vi "DEMO.vi"(8 "errin":errorcluster, 10 "DATA IN":T1) -> (0 "error out":errorcluster)   [LabVIEW 2020]
uses:
  93f8419f-589b-4a81-b62e-70ffcd900bdb.vi
  OP600/SubVI/CheminDeBase.vi
panel:
  out "chaîne concaténée":string
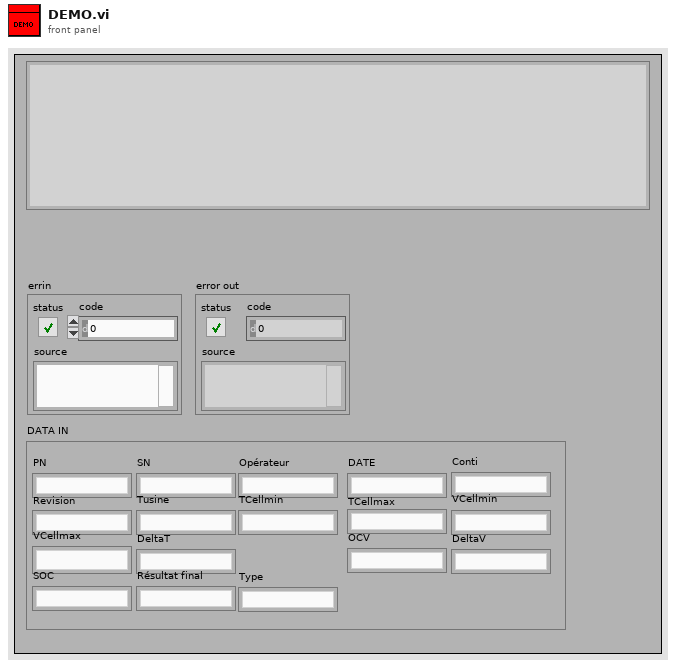
[diagram p1: front panel]
types:
  T1 = cluster{"PN":string, "SN":string, "Opérateur":string, "DATE":string, "Conti":string, "Revision":string, "Tusine":string, "TCellmin":string, "TCellmax":string, "VCellmin":string, "VCellmax":string, "DeltaT":string, "OCV":string, "DeltaV":string, "SOC":string, "Résultat final":string, "Type":string}
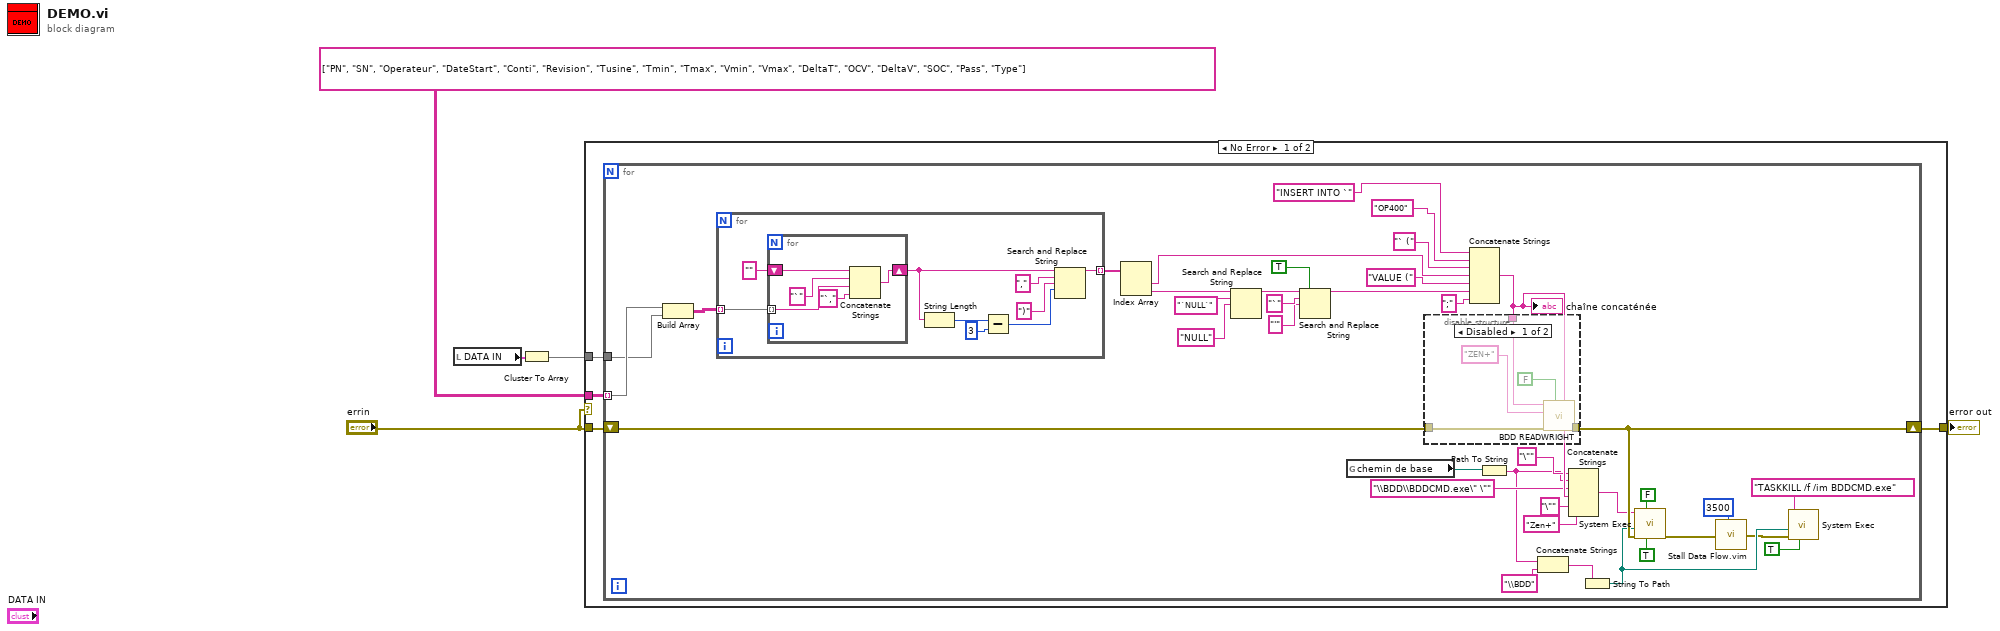
[diagram p0: block diagram]
diagram:
  n1 = local read "DATA IN"() -> (w1:T1)
  n2 = Cluster To Array(cluster=w1) -> (array=w2:string[])
  n3 = case shown="No Error" "errin" {
    tunnel: "errin" -> [w9 w67]
    tunnel: [w8 w67] -> w5
    tunnel: string[][] [["PN", "SN", "Operateur", "DateStart", "Conti", "Revision", "Tusine", "Tmin", "Tmax", "Vmin", "Vmax", "DeltaT", "OCV", "DeltaV", "SOC", "Pass", "Type"]] -> [w7 _]
    tunnel: w2 -> [w6 _]
    frame No Error {
      n4 = for {
        shift-right: [w28] -> w8
        shift-left: w9 -> [w32]
        tunnel: w7 -> [w31] mode=indexing
        tunnel: w6 -> [w30]
        n5 = Build Array(w31, w30) -> (w47:string[][])
        n6 = for {
          tunnel: [w53] -> w33 mode=indexing
          tunnel: w47 -> [w61] mode=indexing
          n7 = for {
            shift-right: [w64] -> w54
            shift-left: "" -> [w63]
            tunnel: w61 -> [w62] mode=indexing
            n8 = Concatenate Strings(w63, "`" ("string"), w62, "`," ("string")) -> (w64:string)
          }
          n9 = String Length(string=w54) -> (length=w59:i32)
          n10 = Subtract(x=w59, y=3) -> (x-y=w57:i32)
          n11 = Search and Replace String(input string=w54, search string=",", replace string=")" ("replace string (\"\")"), offset=w57) -> (result string=w53:string)  [unwired: 4 in, 3 out]
        }
        n12 = Index Array(array=w33) -> (element #1=w43:string, element #2=w44:string)  [unwired: 2 in]
        n13 = Search and Replace String(input string=w44, search string="`NULL`", replace string="NULL" ("replace string (\"\")")) -> (result string=w45:string)  [unwired: 5 in, 3 out]
        n14 = Search and Replace String(replace all?=TRUE ("replace all? (F)"), input string=w45, search string="`", replace string="'" ("replace string (\"\")")) -> (result string=w46:string)  [unwired: 4 in, 3 out]
        n15 = global read "CheminDeBase.vi" "chemin de base"() -> (w15:path)
        n16 = Concatenate Strings("INSERT INTO `" ("string"), "OP400", "` (" ("string"), w43, "VALUE (" ("string"), w46, ";" ("string")) -> (w29:string)
        "chaîne concaténée" <- w29
        n17 = disable-structure shown="Disabled" {
          disable-tunnel: w29 -> [w52 _]
          disable-tunnel: w32 -> [w51 _]
          disable-tunnel: [w50 _] -> w28
          frame Disabled {
            n18 = call "BDD READWRIGHT.vi"("Read?"=FALSE, "errin"=w51, "DSN name"="ZEN+", "Instruction"=w52) -> ("error out"=w50:errorcluster)  [unwired: 6 in, 1 out]
          }
          frame Enabled {
          }
        }
        n19 = Path To String(path=w15) -> (string=w19:string)
        n20 = Concatenate Strings(w19, "\\BDD" ("chaîne")) -> (w17:string)
        n21 = Concatenate Strings("\"" ("chaîne"), w19, "\\BDD\\BDDCMD.exe\" \"" ("string"), w29, "\"" ("string"), "Zen+" ("string")) -> (w26:string)
        n22 = String To Path(string=w17) -> (path=w16:path)
        n23 = call <vilib>:"System Exec.vi"("run minimized? (F)"=TRUE, "wait until completion? (T)"=FALSE, "error in (no error)"=w28, "working directory"=w16, "command line"=w26) -> ("error out"=w27:errorcluster)  [unwired: 3 in, 3 out]
        n24 = call "Stall Data Flow.vim"("value in"=w27, "milliseconds to wait"=u32 3500) -> ("value out"=w13:errorcluster)  [unwired: 1 out]
        n25 = call <vilib>:"System Exec.vi"("run minimized? (F)"=TRUE, "error in (no error)"=w13, "working directory"=w16, "command line"="TASKKILL /f /im BDDCMD.exe") -> ()  [unwired: 4 in, 4 out]
      }
    }
    frame Error {
    }
  }
  "error out" <- w5
